vi "ReadConnInfo.vi"(8 "error in (no error)":errorcluster) -> (0 "error out":errorcluster, 2 "found":bool, 3 "connection info":T1={"ClientName"="", "TransceiverHost"="", "TransceiverPort"=6342, "Password"=""})   [LabVIEW 2017, in "ServerComm.lvlib"]
uses:
  <vilib>/addons/InsightCM/Devices/Shared/Common/ServerComm/ServerComm.lvlib
  <vilib>/addons/InsightCM/MessageBus/Base/controls/ConnectionInfo.ctl
  <vilib>/addons/InsightCM/Utilities/GlobalConfiguration/GlobalConfiguration.lvlib
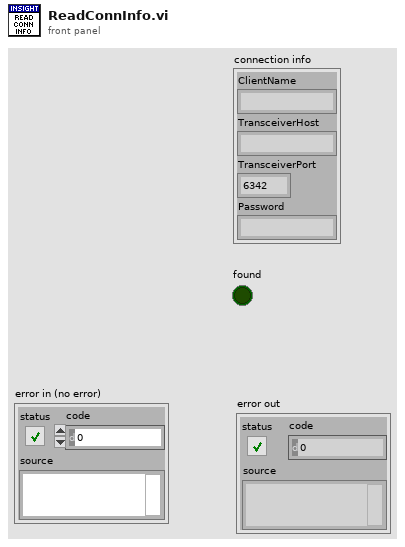
[diagram p1: front panel]
types:
  T1 = typedef "ConnectionInfo.ctl" = cluster{"ClientName":string, "TransceiverHost":string, "TransceiverPort":u16, "Password":string}
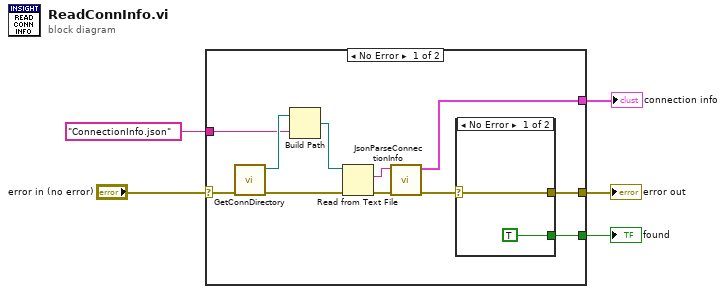
[diagram p0: block diagram]
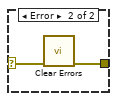
[diagram p2: hidden frame]
diagram:
  n1 = case shown="No Error" "error in (no error)" {
    selector: "error in (no error)" -> [w12 w21]
    tunnel: [w15 w21] -> w4
    tunnel: [w16 _] -> w3
    tunnel: [w13 _] -> w2
    tunnel: "ConnectionInfo.json" ("json object") -> [w7 _]
    frame No Error {
      n2 = call <vilib>:"GetConnDirectory.vi"("error in (no error)"=w12) -> ("error out"=w10:errorcluster, "application directory"=w8:path)  [unwired: 9 in]
      n3 = Build Path(base path=w8, name or relative path=w7) -> (appended path=w11:path)
      n4 = Read from Text File(file (use dialog)=w11, error in=w10) -> (text=w6:string, error out=w9:errorcluster)  [unwired: 2 in, 2 out]
      n5 = call <vilib>:"JsonParseConnectionInfo.vi"("error in (no error)"=w9, "JSON string"=w6) -> ("error out"=w14:errorcluster, "connection info"=w16:T1)  [unwired: 8 in]
      n6 = case shown="No Error" w14 {
        selector: w14 -> [w18 w19]
        tunnel: [w18 w20] -> w15
        tunnel: [TRUE _] -> w13
        frame No Error {
        }
        frame Error {
          n7 = call <vilib>:"Clear Errors.vi"("error in (no error)"=w19) -> ("error out"=w20:errorcluster)  [unwired: 5 in, 1 out]
        }
      }
    }
    frame Error {
    }
  }
  "error out" <- w4
  "connection info" <- w3
  "found" <- w2
